vi "Check.vi"(0 "Uno in":refnum<class "Uno.lvclass">, 11 "error in":errorcluster) -> (4 "Uno out":refnum<class "Uno.lvclass">, 6 "run":bool, 10 "open direction":T1, 12 "open count":i16, 13 "friendly zone":bool, 14 "open coord":cluster{"X":i32, "Y":i32}, 15 "error out":errorcluster)   [LabVIEW 2020, in "Uno.lvclass"]
uses:
  Uno.lvclass
  Type Defs/Direction Enum.ctl
  Uno.lvclass/Uno.ctl
  Type Defs/SB Type Defs.lvlib
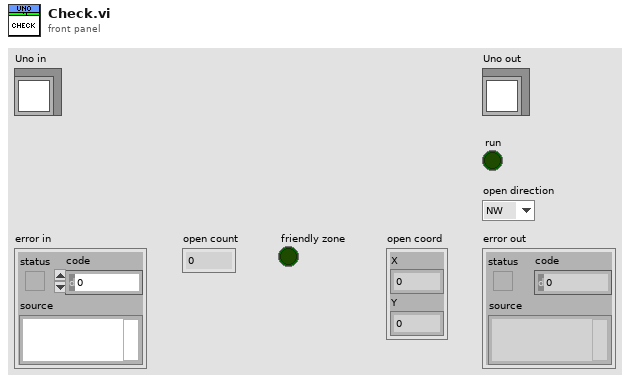
[diagram p1: front panel]
types:
  T1 = typedef "SB Type Defs.lvlib/Direction Enum.ctl" = enum16{"NW", "N", "NE", "E", "SE", "S", "SW", "W"}
  T2 = typedef "Uno.lvclass/Group Data.ctl" = cluster{"our positions":u8[][]}
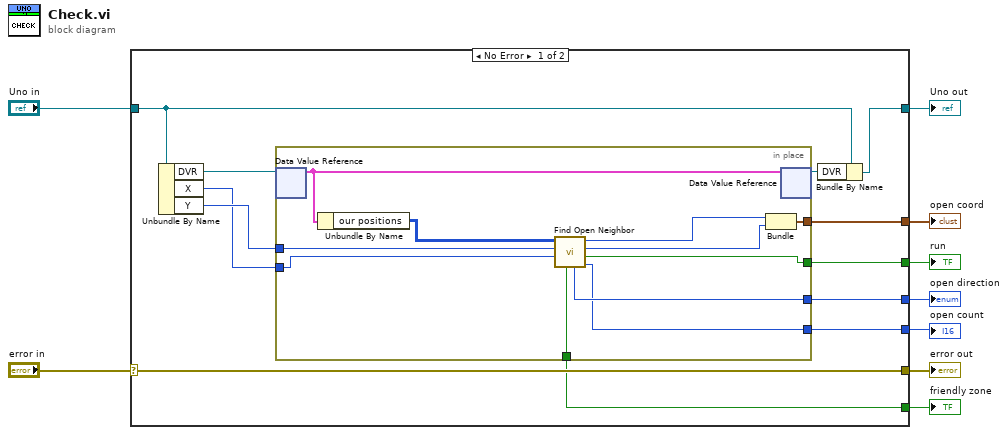
[diagram p0: block diagram]
diagram:
  n1 = case shown="No Error" "error in" {
    selector: "error in" -> [w12 w34]
    tunnel: [w12 w34] -> w8
    tunnel: [w20 w33] -> w6
    tunnel: "Uno in" -> [w21 w33]
    tunnel: [w15 _] -> w5
    tunnel: [w14 _] -> w4
    tunnel: [w13 _] -> w3
    tunnel: [w11 _] -> w2
    tunnel: [w10 _] -> w1
    frame No Error {
      n2 = Unbundle By Name(w21) -> ("DVR"=w18:refnum<data-value>, "X"=w16:i32, "Y"=w17:i32)
      n3 = in-place {
        in-place-border: w17 -> [w30]
        in-place-border: w16 -> [w31]
        in-place-border: [w29] -> w15
        in-place-border: [w28] -> w14
        in-place-border: [w27] -> w13
        in-place-border: [w23] -> w11
        in-place-border: [w22] -> w10
        n4 = in-place-dvr #1(w18) -> (w32:T2)  [unwired: 1 out]
        n5 = Unbundle By Name(w32) -> ("our positions"=w24:u8[][])
        n6 = call "Find Open Neighbor.vi"("X"=w31, "Y"=w30, "our positions"=w24) -> ("open count"=w23:i16, "open?"=w29:bool, "open y"=w26:i32, "open x"=w25:i32, "open direction"=w28:T1, "friendly zone"=w22:bool)  [unwired: 3 in]
        n7 = Bundle("open x"=w25, "open y"=w26) -> (w27:cluster{"open x":i32, "open y":i32})  [unwired: 1 in]
        n8 = in-place-dvr #1(w32) -> (w19:refnum<data-value>)  [unwired: 1 out]
      }
      n9 = Bundle By Name(cluster=w21, "DVR"=w19) -> (w20:refnum<class "Uno.lvclass">)
    }
    frame Error {
    }
  }
  "error out" <- w8
  "Uno out" <- w6
  "run" <- w5
  "open direction" <- w4
  "open coord" <- w3
  "open count" <- w2
  "friendly zone" <- w1
